vi "DSF file to data.vi"(8 "error in (no error)":errorcluster, 11 "configuration file cluster in":T1) -> (0 "error out":errorcluster, 2 "configuration data cluster out":T9, 3 "configuration file cluster out":T1)   [LabVIEW 2017, in "DSF Configuration API v1.0.0.lvlib"]
uses:
  DSF Configuration API v1.0.0.lvlib
  Controls/dsf configuration file/1.0.0/dsf configuration.ctl
  Controls/dsf configuration file/1.0.0/version.ctl
  Controls/dsf configuration file/1.0.0/dsf plugin.ctl
  Controls/dsf configuration file/1.0.0/dsf timing.ctl
  Controls/dsf configuration file/1.0.0/dsf group.ctl
  Controls/dsf configuration file/1.0.0/dsf transfer.ctl
  Controls/dsf configuration file/1.0.0/dsf channel.ctl
  Controls/dsf configuration file/1.0.0/dsf settings.ctl
  Controls/dsf configuration data/1.0.0/dsf configuration.ctl
  Controls/dsf configuration data/1.0.0/version.ctl
  Controls/dsf configuration data/1.0.0/dsf plugin.ctl
  Controls/dsf configuration data/1.0.0/dsf timing.ctl
  Controls/dsf configuration data/1.0.0/dsf group.ctl
  Controls/dsf configuration data/1.0.0/dsf transfer.ctl
  Controls/dsf configuration data/1.0.0/dsf channel.ctl
  Controls/dsf configuration data/1.0.0/dsf settings.ctl
  Controls/dsf configuration data/1.0.0/dsf configuration data v1.0.0.lvlib
  Controls/dsf configuration file/1.0.0/dsf configuration file v1.0.0.lvlib
panel:
  # "dsf\nfile"
  # "dsf\ncfg"
  # "dsf\nfile"
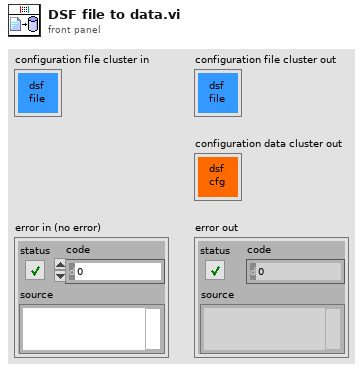
[diagram p1: front panel]
types:
  T1 = typedef "dsf configuration file v1.0.0.lvlib/dsf configuration.ctl" = cluster{"dsf":T2, "configuration":T2, "plugins":T3[], "groups":T5[], "transfers":T6[], "channels":T7[], "settings":T8[]}
  T2 = typedef "dsf configuration file v1.0.0.lvlib/version.ctl" = cluster{"major":u32, "minor":u32, "fix":u32, "build":string}
  T3 = typedef "dsf configuration file v1.0.0.lvlib/dsf plugin.ctl" = cluster{"id":string, "values":cluster{"type":string, "timing":T4, "group ids":string[], "settings id":string}}
  T4 = typedef "dsf configuration file v1.0.0.lvlib/dsf timing.ctl" = cluster{"decimation":i32, "offset":i32}
  T5 = typedef "dsf configuration file v1.0.0.lvlib/dsf group.ctl" = cluster{"id":string, "values":cluster{"direction":i32, "timing":T4, "transfer ids":string[], "settings id":string}}
  T6 = typedef "dsf configuration file v1.0.0.lvlib/dsf transfer.ctl" = cluster{"id":string, "values":cluster{"byte order":i32, "channel ids":string[], "settings id":string}}
  T7 = typedef "dsf configuration file v1.0.0.lvlib/dsf channel.ctl" = cluster{"id":string, "values":cluster{"count":i32, "offset":i32, "data type":i32, "resource path":string, "settings id":string}}
  T8 = typedef "dsf configuration file v1.0.0.lvlib/dsf settings.ctl" = cluster{"id":string, "values":cluster{"key":string, "value":string}[]}
  T9 = typedef "dsf configuration data v1.0.0.lvlib/dsf configuration.ctl" = cluster{"dsf schema version":T10, "configuration version":T10, "plugins":T11[]}
  T10 = typedef "dsf configuration data v1.0.0.lvlib/version.ctl" = cluster{"major":u32, "minor":u32, "fix":u32, "build":string}
  T11 = typedef "dsf configuration data v1.0.0.lvlib/dsf plugin.ctl" = cluster{"id":string, "values":cluster{"type":string, "timing":T12, "groups":T13[], "settings":T16}}
  T12 = typedef "dsf configuration data v1.0.0.lvlib/dsf timing.ctl" = cluster{"decimation":i32, "offset":i32}
  T13 = typedef "dsf configuration data v1.0.0.lvlib/dsf group.ctl" = cluster{"id":string, "values":cluster{"direction":i32, "timing":T12, "transfers":T14[], "settings":T16}}
  T14 = typedef "dsf configuration data v1.0.0.lvlib/dsf transfer.ctl" = cluster{"id":string, "values":cluster{"byte order":i32, "channels":T15[], "settings":T16}}
  T15 = typedef "dsf configuration data v1.0.0.lvlib/dsf channel.ctl" = cluster{"id":string, "values":cluster{"count":i32, "offset":i32, "data type":i32, "resource path":string, "settings":T16}}
  T16 = typedef "dsf configuration data v1.0.0.lvlib/dsf settings.ctl" = cluster{"id":string, "values":cluster{"key":string, "value":string}[]}
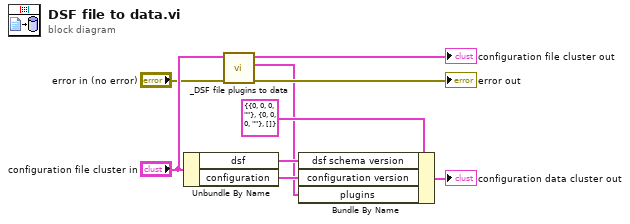
[diagram p0: block diagram]
diagram:
  n1 = Unbundle By Name("configuration file cluster in") -> ("dsf"=w8:T2, "configuration"=w7:T2)
  n2 = call "_DSF file plugins to data.vi"("error in (no error)"="error in (no error)", "configuration file cluster in"="configuration file cluster in") -> ("error out"=→"error out":errorcluster, "plugins"=w2:T11[], "configuration file cluster out"=→"configuration file cluster out":T1)  [unwired: 7 in]
  n3 = Bundle By Name(cluster=T9 {"dsf schema version"={"major"=0, "minor"=0, "fix"=0, "build"=""}, "configuration version"={"major"=0, "minor"=0, "fix"=0, "build"=""}, "plugins"=[]} ("configuration data cluster out"), "dsf schema version"=w8, "configuration version"=w7, "plugins"=w2) -> (→"configuration data cluster out":T9)
